vi "Init Events.vi"(8 "error in (no error)":errorcluster, 11 "InsertionPalettePanel in":refnum<class "InsertionPalettePanel.lvclass">) -> (0 "error out":errorcluster, 3 "InsertionPalettePanel out":refnum<class "InsertionPalettePanel.lvclass">)   [LabVIEW 2020, in "TSnax UI.lvlib" / "InsertionPalettePanel.lvclass"]
uses:
  InsertionPalettePanel.lvclass
  InsertionPalettePanel.lvclass/InsertionPalettePanel.ctl
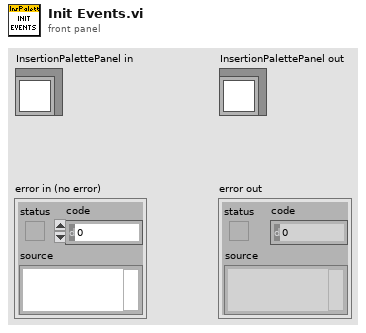
[diagram p1: front panel]
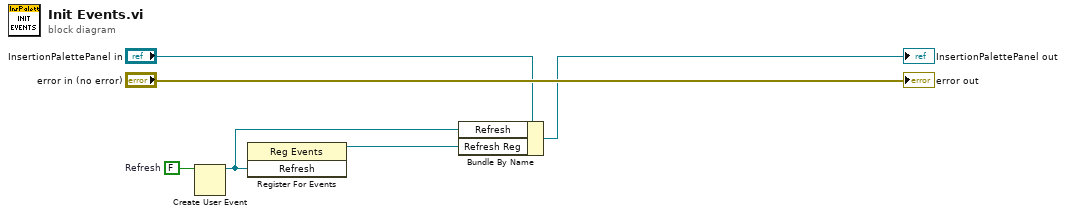
[diagram p0: block diagram]
diagram:
  w4 = FALSE  # Refresh
  n1 = Create User Event(user event datatype=w4) -> (user event=w2:refnum<user-event>)  [unwired: 1 in, 1 out]
  n2 = register-events(w2) -> (reference out=w1:refnum<event-registration>)  [unwired: 2 in, 1 out]
  n3 = Bundle By Name(cluster="InsertionPalettePanel in", "Refresh"=w2, "Refresh Reg"=w1) -> (→"InsertionPalettePanel out":refnum<class "InsertionPalettePanel.lvclass">)
  "error out" <- "error in (no error)"
